vi "Do.vi"(8 "error in":errorcluster, 10 "Actor in":refnum<class "Actor.lvclass">, 11 "Send Shutdown MSG":refnum<class "Send Shutdown MSG.lvclass">) -> (0 "error out":errorcluster, 2 "Actor out":refnum<class "Actor.lvclass">)   [LabVIEW 2017, in "Controller.lvlib" / "Send Shutdown MSG.lvclass"]
doc: "(<B>Filename</B>: Actor Framework.lvlib:Message.lvclass:Do.vi)\n\nDefines what a message does when it is received by an actor. Generally, a message instructs an actor to invoke one of its methods. By default, this method does nothing. A child class must override it to define behavior. Create a child class by using the Actor Framework Message Maker dialog box."
uses:
  Send Shutdown MSG.lvclass
  <vilib>/ActorFramework/Actor/Actor.lvclass
  gController.lvclass
  C:/Program Files (x86)/National Instruments/LabVIEW 2017/vi.lib/MSR Consulting, LLC/General Reuse/SuperActor/SuperActor.lvclass
  C:/Program Files (x86)/National Instruments/LabVIEW 2017/vi.lib/ActorFramework/Actor/Actor.lvclass
  <vilib>/MSR Consulting, LLC/General Reuse/SuperActor/SuperActor.lvclass/SuperActor.ctl
  <vilib>/MSR Consulting, LLC/General Reuse/SuperActor/Read CVT Session.vi
  <vilib>/MSR Consulting, LLC/General Reuse/SuperActor/Messages/Shutdown/Send Shutdown MSG.lvclass
  <vilib>/MSR Consulting, LLC/General Reuse/Session APIs/_Session Fwk/Session - Root.lvclass
  <vilib>/MSR Consulting, LLC/General Reuse/Session APIs/CVT/CVT.lvclass
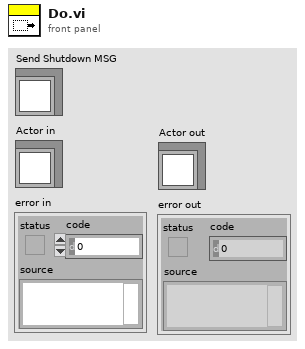
[diagram p1: front panel]
types:
  T1 = typedef "Session - Root.lvclass/Session Handle.ctl" = refnum<data-value>
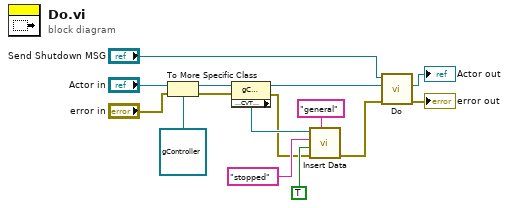
[diagram p0: block diagram]
diagram:
  n1 = To More Specific Class(target class=refnum<class "gController.lvclass"> refnum ("Controller.lvlib:gController"), reference="Actor in", error in="error in") -> (specific class reference=w11:refnum<class "gController.lvclass">, error out=w3:errorcluster)
  n2 = property class="gController"(reference=w11, error in=w3) -> (reference out=w5:refnum<class "gController.lvclass">, error out=w1:errorcluster, "Accessors:CVT Session"=w10:T1)
  n3 = call <vilib>:"Insert Data.vi"("Group"="general", "error in"=w1, "Data"=TRUE, "tag"="stopped", "CVT Session In"=w10) -> ("error out"=w4:errorcluster)  [unwired: 5 in, 1 out]
  n4 = call-parent "Do.vi"("error in"=w4, "Actor in"=w5, "Send Shutdown MSG"="Send Shutdown MSG") -> ("error out"=→"error out":errorcluster, "Actor out"=→"Actor out":refnum<class "Actor.lvclass">)  [unwired: 7 in]
